vi "EllipseDetection.vi"(0 "Motor an?":bool=TRUE, 1 "Sweep":dbl[](array[numeric])=array[10000 elements], 2 "Winkel_ende":dbl=0.982793723247329, 4 "Sequenz length us":i32=10000, 5 "x_Ellipse":i32=110, 6 "Schrittweite (°)":dbl=1.8 min=0.8999999761581421 max=180.0 step=0.1) -> (7 "Gaparray":dbl[](array[numeric])=[0.0, 0.0, 0.0, 0.0, 0.0, 0.0, 0.0, 0.0, 31.78266847459895, 71.77897962111933, 69.81599676332462, 70.62742631416654, 70.53536343963606, 70.80018094433717, 71.92808960208231, 73.2443285987772, 73.64080618998037, 74.55555718210849], 8 "Max. Index":i32=17, 10 "Maximale Gap":dbl=74.55555718210849, 11 "Wahrscheinlichkeit*Apulitude":dbl[](array[numeric])=[0.0, 0.0, 0.0, 0.0, 0.0, 0.0, 0.0, 0.0, 4.587844159843566e-180, 5.197567004295835, 0.18885512712583885, 1.8492331967600593, 3.0203550412227926, 8.509948855746485, 82.25615517554286, 367.57708439761143, 518.7343556046903, 579.1392161246325], 12 "IR with theshold":dbl[][](graph), 13 "Maximale Gap gefunde?":bool, 14 "Welche Mikrofon arbeitet":tag="Dev2/ai2", 15 "Welche LS arbeitet":i32=4, 16 "Abstatnd":dbl, 17 "Peak Locations":dbl[](array[numeric])=[1600.9324970830344, 1675.4880542651429], 18 "Gap":dbl=74.55555718210849, 19 "Wahrscheinlichkeit":dbl=0.25453954610461715)   [LabVIEW 2014]
uses:
  <vilib>/Analysis/NI_AALBase.lvlib
  <vilib>/Analysis/3filter.llb/Filter Passband Type.ctl
  <vilib>/Analysis/NI_AALPro.lvlib
  <vilib>/Analysis/2dsp.llb/1D Cross Correlation (DBL).vi
  <vilib>/Analysis/3filter.llb/Butterworth Filter (DBL).vi
  <vilib>/Instr/_visa.llb/VISA Configure Serial Port (Instr).vi
panel:
  in  "Registerkarte":T1(tab)=enum."Gap & Wahrscheinlickeit"
  out "Sweep-signal":dbl[](graph)
  out "Anzahl\nMessungen":dbl=18.21266317958185
  in  "Motorwahl":string(combo)="0"
  in  "Stromstärke in mA / 10":u8=40 max=200 step=1
  in  "Schrittgeschwindigkeit":u8=20
  out "time at begin":timestamp=timestamp(3560686964.139921 s since 1904-01-01)
  in  "RN-Motor - RS232":refnum<visa-resource-name>="COM5"
  out "Active Speaker":bool[](array[boolean])=[FALSE, FALSE, FALSE, TRUE, FALSE, FALSE, FALSE, FALSE, FALSE, FALSE, FALSE, FALSE, FALSE, FALSE]
  out "drehrichtung":u8=1
  out "Rohdaten Mic_1":dbl[](graph)
  in  "begin signal":dbl=10000.0
  out "Korreliertes Signal mit richtigem Anfang -M1":dbl[](graph)
  out "Mit Sweep korreliert 1":dbl[](graph)
  in  "Noise Level":dbl=4.0
  in  "RMS miutiplication factor":dbl=3.0
  in  "MaxtPeak miltiplication factor":dbl=7.0
  in  "Grenz Ampulitude":dbl=80.0
  in  "StandardGap":dbl=75.0
  in  "Sigma in Prozent":dbl=2.0
  out "t_2":dbl=1675.4880542651429
  out "t_1":dbl=1600.9324970830344
  out "W * A":dbl=579.1392161246325
  out "Wahrschwinlichkeitsarray":dbl[](array[numeric])=[0.0, 0.0, 0.0, 0.0, 0.0, 0.0, 0.0, 0.0, 1.4779650144959823e-181, 0.026517429714331527, 0.0006779892682999901, 0.003798460831457268, 0.0031702188135415243, 0.005278750347818211, 0.032665581582708055, 0.1340721173746843, 0.17641101202507742, 0.25453954610461715]
  out "Max. Wert":dbl=579.1392161246325
  out "W *A-1":dbl[](array[numeric])=[0.0, 0.0, 0.0, 0.0, 0.0, 0.0, 0.0, 0.0, 4.587844159843566e-180, 5.197567004295835, 0.18885512712583885, 1.8492331967600593, 3.0203550412227926, 8.509948855746485, 82.25615517554286, 367.57708439761143, 518.7343556046903, 579.1392161246325]
  out "GapArray -1":dbl[](array[numeric])=[0.0, 0.0, 0.0, 0.0, 0.0, 0.0, 0.0, 0.0, 31.78266847459895, 71.77897962111933, 69.81599676332462, 70.62742631416654, 70.53536343963606, 70.80018094433717, 71.92808960208231, 73.2443285987772, 73.64080618998037, 74.55555718210849]
  out "t1 Array":dbl[](array[numeric])=[0.0, 0.0, 0.0, 0.0, 0.0, 0.0, 0.0, 0.0, 1194.5330720667082, 1555.0449407198062, 1560.1513249404838, 1564.0418298861218, 1569.529647486898, 1575.4886309745948, 1581.693370955709, 1587.7292742626732, 1594.4280385114012, 1600.9324970830344]
  out "x_Ellipse>100":bool=TRUE
  # "0=links\n1=rechts"
  # "M1: ai2\nM2: ai1"
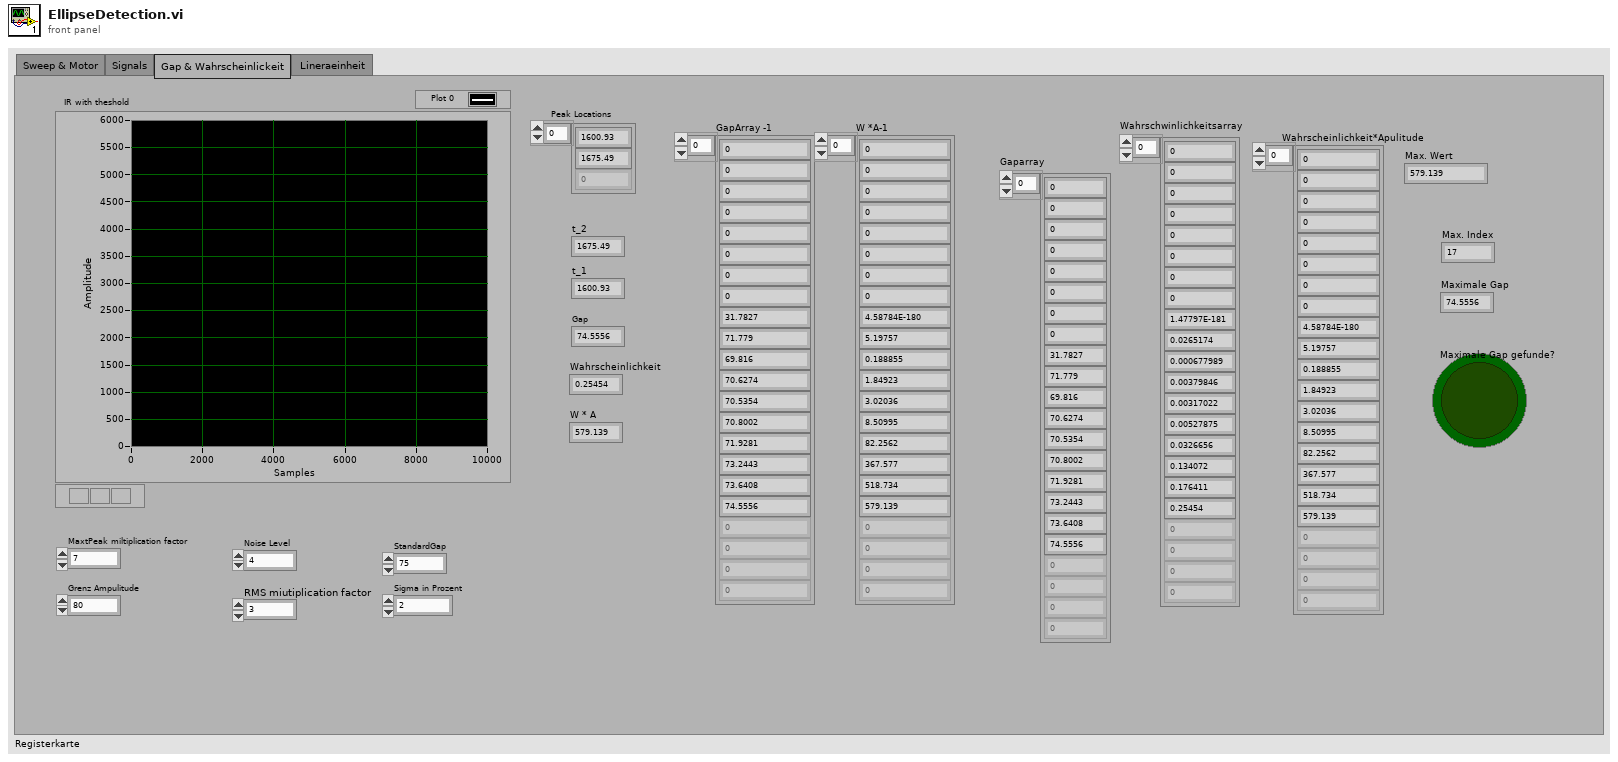
[diagram p1: front panel]
types:
  T1 = enum32{"Sweep & Motor", "Signals", "Gap & Wahrscheinlickeit", "Lineraeinheit "}
  T2 = cluster{"VISA resource name out":refnum<visa-resource-name>, "Motorwahl":string, "Schrittweite (°)":dbl, "error out":errorcluster}
  T3 = cluster{"VISA resource name out":refnum<visa-resource-name>, "Gesendeter Code":string, "Schrittweite (°)":dbl, "error out":errorcluster}
  T4 = typedef "NI_AALBase.lvlib/Filter Passband Type.ctl" = enum32{"Lowpass", "Highpass", "Bandpass", "Bandstop"}
  T5 = cluster{"VISA resource name out":refnum<visa-resource-name>, "Gesendeter Code":string, "error out":errorcluster}
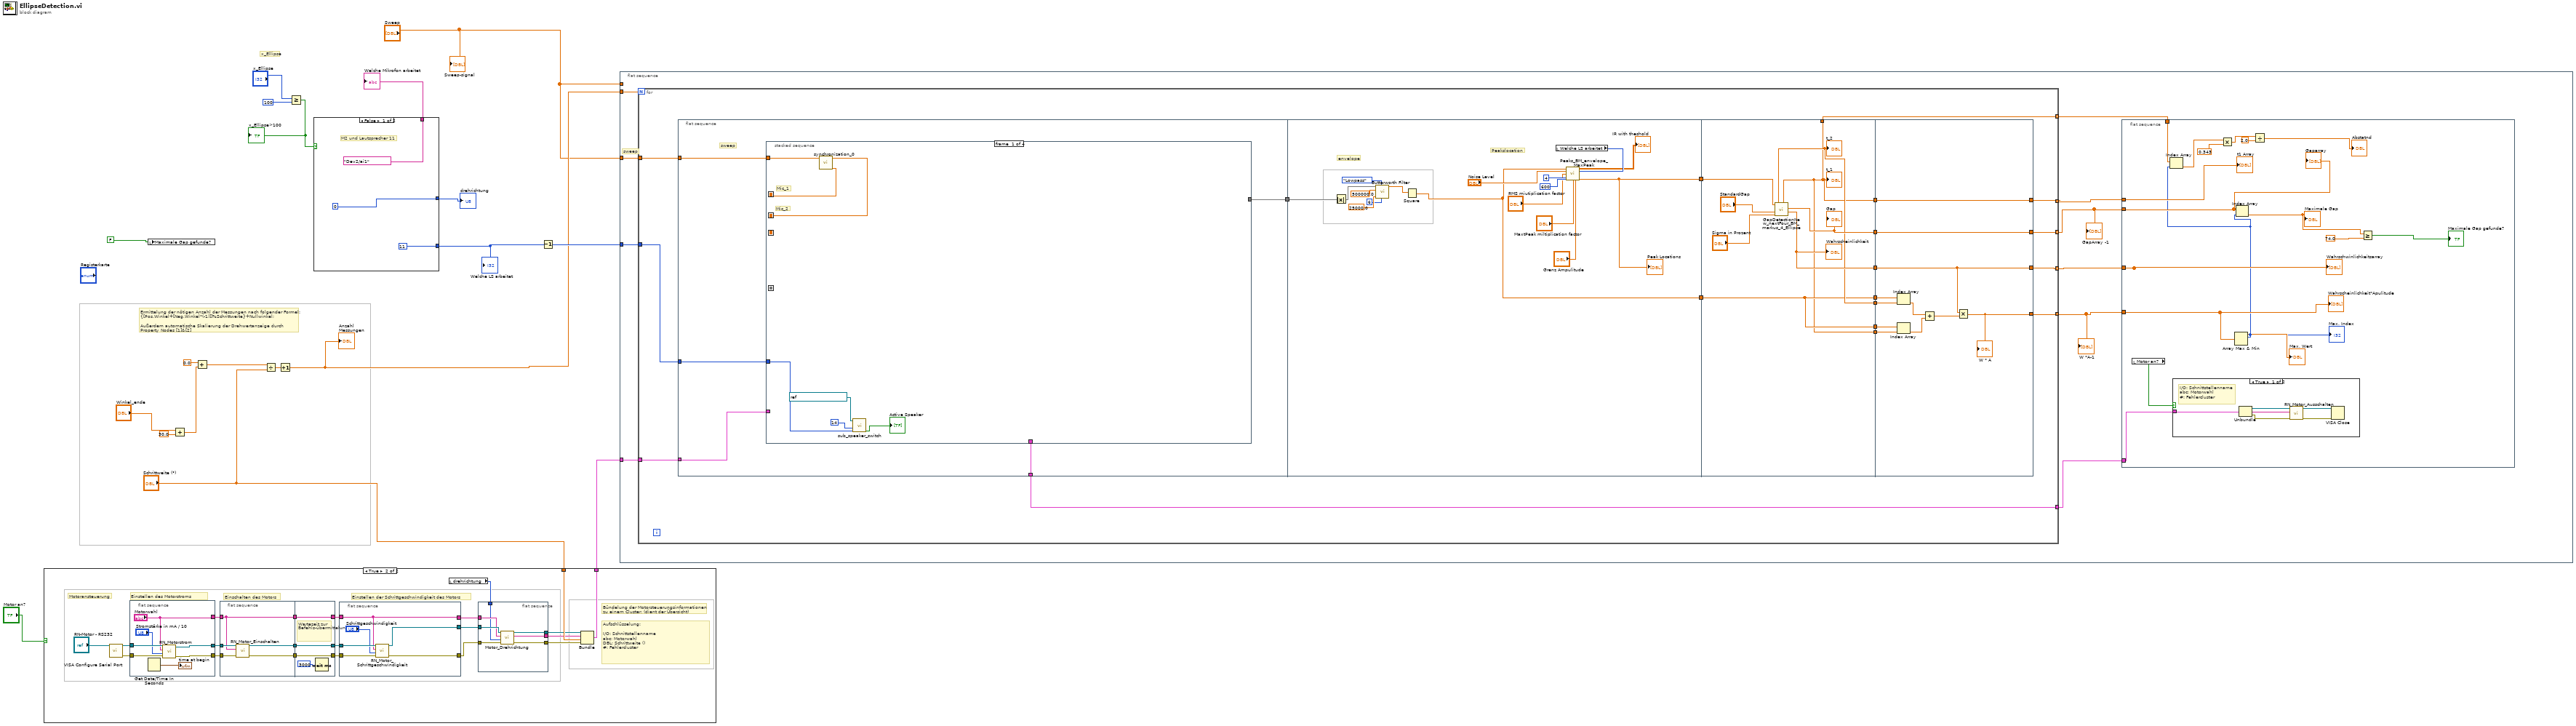
[diagram p0: block diagram]
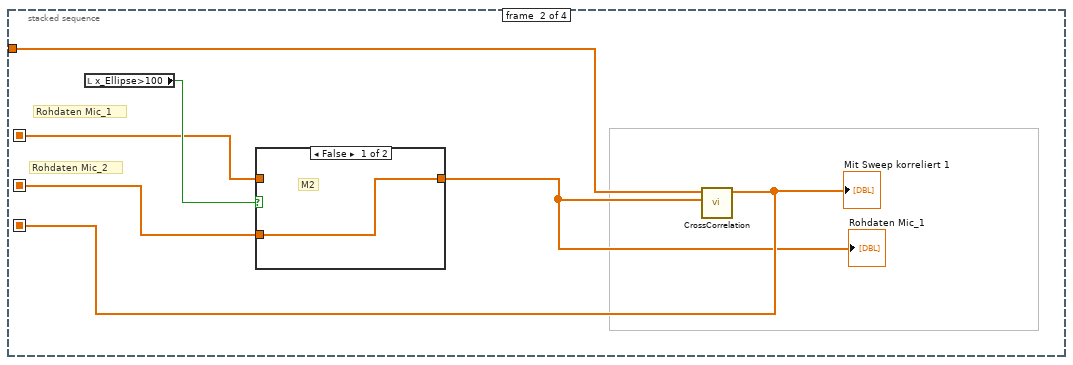
[diagram p3: hidden frame]
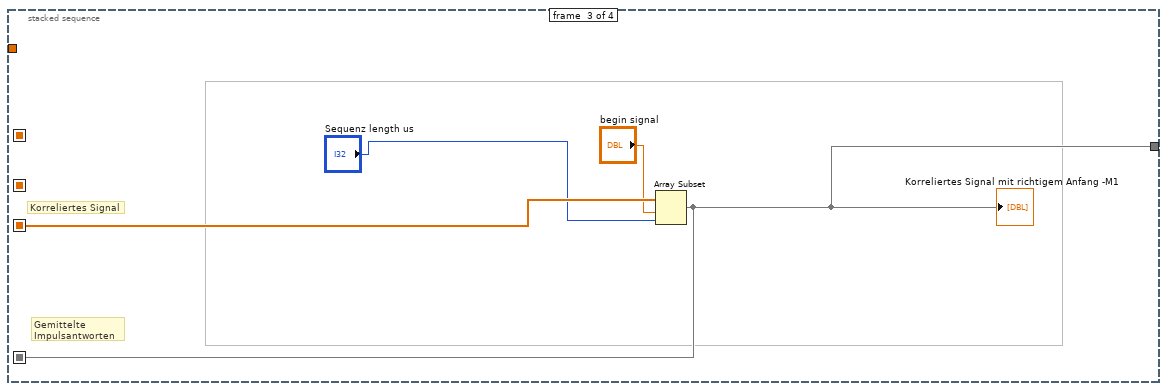
[diagram p5: hidden frame]
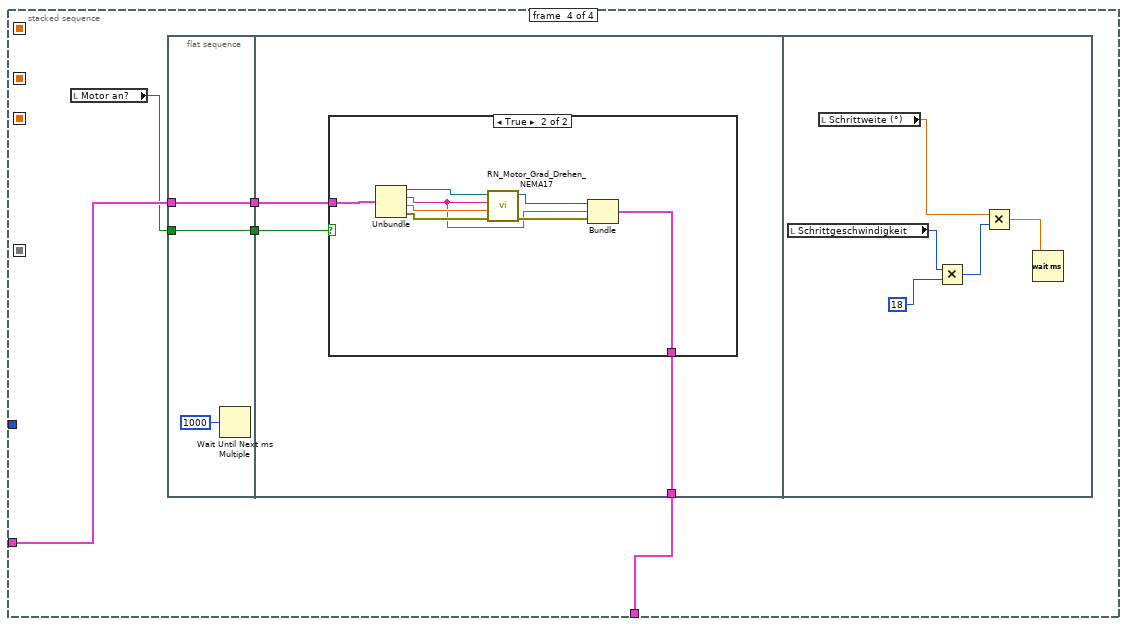
[diagram p6: hidden frame]
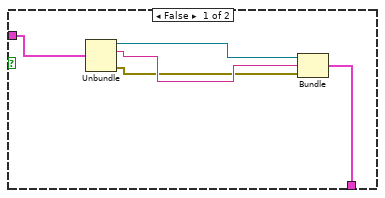
[diagram p7: hidden frame]
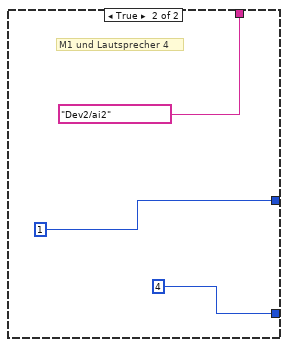
[diagram p8: hidden frame]
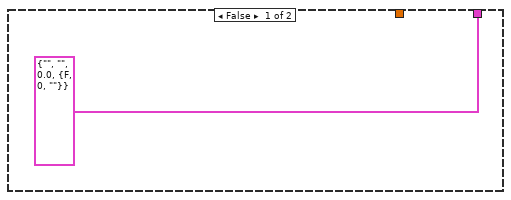
[diagram p9: hidden frame]
diagram:
  # "x_Ellipse"
  # "Ermittelung der nötigen Anzahl der Messungen nach folgender Formel:\n{[Pos.Winkel+[Neg.Winkel*(-1)]]%Schrittweite}+Nullwinkel;\n\nAußerdem automatische Skalierung der Drehwertanzeige durch \nProperty Nodes [1]&[2]"
  n1 = case shown="True" "Motor an?" {
    tunnel: "Schrittweite (°)" -> [_ w29]
    tunnel: [T2 {"VISA resource name out"="", "Motorwahl"="", "Schrittweite (°)"=0.0, "error out"={"status"=FALSE, "code"=0, "source"=""}} ("output cluster") w28] -> w17
    frame False {
    }
    frame True {
      # "Aufschlüsselung:\n\nI/O: Schnittstellenname\nabc: Motorwahl \nDBL: Schrittweite ()\n#: Fehlercluster"
      # "Bündelung der Motorsteuerungsinformationen \nzu einem Cluster: (dient der Übersicht)"
      # "Einstellen der Schrittgeschwindigkeit des Motors"
      # "Einschalten des Motors"
      # "Einstellen des Motorstroms"
      # "Motoransteuerung"
      n2 = call-poly "VISA Configure Serial Port"("VISA resource name"="RN-Motor - RS232") -> ("VISA resource name out"=w37:refnum<visa-resource-name>, "error out"=w36:errorcluster)  [unwired: 13 in]
      n3 = flat-sequence {
        tunnel: w37 -> [w70]
        tunnel: w36 -> [w69]
        tunnel: [w67] -> w35
        tunnel: [w66] -> w34
        tunnel: ["Motorwahl"] -> w30
        frame #0 {
          n4 = Get Date/Time In Seconds() -> (seconds since 1Jan1904=→"time at begin":timestamp)
          n5 = call "RN_Motorstrom.vi"("error in"=w69, "Stromstärke in mA / 10"="Stromstärke in mA / 10", "Motorwahl"="Motorwahl", "VISA resource name in"=w70) -> ("error out"=w66:errorcluster, "VISA resource name out"=w67:refnum<visa-resource-name>)  [unwired: 3 in, 1 out]
        }
      }
      n6 = flat-sequence {
        tunnel: w35 -> [w59]
        tunnel: w34 -> [w58]
        tunnel: w30 -> [w55]
        tunnel: [w57] -> w41
        tunnel: [w56] -> w40
        tunnel: [w55] -> w39
        tunnel: [w62] -> w32
        tunnel: [w63] -> w33
        tunnel: w41 -> [w63]
        tunnel: w40 -> [w62]
        tunnel: [w60] -> w31
        tunnel: w39 -> [w60]
        frame #0 {
          n7 = call "RN_Motor_Einschalten.vi"("error in"=w58, "Motorwahl"=w55, "VISA resource name in"=w59) -> ("error out"=w56:errorcluster, "VISA resource name out"=w57:refnum<visa-resource-name>)  [unwired: 3 in, 2 out]
        }
        frame #1 {
          # "Wartezeit zur Befehls-übermittelung"
          n8 = Wait (ms)(milliseconds to wait=u32 3000) -> ()  [unwired: 1 out]
        }
      }
      n9 = flat-sequence {
        tunnel: w33 -> [w54]
        tunnel: w32 -> [w53]
        tunnel: [w51] -> w27
        tunnel: w31 -> [w50]
        tunnel: [w50] -> w23
        tunnel: [w49] -> w25
        frame #0 {
          n10 = call "RN_Motor_Schrittgeschwindigkeit.vi"("error in"=w53, "Schrittgeschwindigkeit"="Schrittgeschwindigkeit", "Motorwahl"=w50, "VISA resource name in"=w54) -> ("error out"=w51:errorcluster, "VISA resource name out"=w49:refnum<visa-resource-name>)  [unwired: 3 in, 1 out]
        }
      }
      n11 = local read "drehrichtung"() -> (w21:u8)
      n12 = flat-sequence {
        tunnel: w27 -> [w48]
        tunnel: [w47] -> w26
        tunnel: w25 -> [w46]
        tunnel: [w45] -> w24
        tunnel: w23 -> [w44]
        tunnel: [w43] -> w22
        tunnel: w21 -> [w42]
        frame #0 {
          n13 = call "Motor_Drehrichtung.vi"("error in"=w48, "drehrichtung"=w42, "Motorwahl"=w44, "VISA resource name in"=w46) -> ("error out"=w47:errorcluster, "Gesendeter Code"=w43:string, "VISA resource name out"=w45:refnum<visa-resource-name>)  [unwired: 5 in]
        }
      }
      n14 = Bundle("VISA resource name out"=w24, "Gesendeter Code"=w22, "Schrittweite (°)"=w29, "error out"=w26) -> (w28:T3)  [unwired: 1 in]
    }
  }
  n15 = local write "Maximale Gap gefunde?"(FALSE ("Maximale Gap gefunde?")) -> ()
  n16 = Add(x="Winkel_ende", y=30.0) -> (x+y=w3:dbl)
  n17 = Add(x=0.0, y=w3) -> (x+y=w18:dbl)
  n18 = Divide(x=w18, y="Schrittweite (°)") -> (x/y=w19:dbl)
  n19 = Increment(x=w19) -> (x+1=w8:dbl)
  "Anzahl\nMessungen" <- w8
  n20 = Greater Or Equal?(x="x_Ellipse", y=100) -> (x >= y?=w12:bool)
  "x_Ellipse>100" <- w12
  n21 = case shown="False" w12 {
    tunnel: [11 ("Num of Speakers") 4 ("y")] -> w10
    tunnel: [tag "Dev2/ai1" ("physical channels 2") tag "Dev2/ai2" ("physical channels 2")] -> w13
    tunnel: [0 1] -> w6
    frame False {
      # "M2 und Lautsprecher 11"
    }
    frame True {
      # "M1 und Lautsprecher 4"
    }
  }
  "Welche Mikrofon arbeitet" <- w13
  "Welche LS arbeitet" <- w10
  "drehrichtung" <- w6
  n22 = Decrement(x=w10) -> (x-1=w9:i32)
  n23 = flat-sequence {
    tunnel: w8 -> [w86]
    tunnel: w17 -> [w85]
    tunnel: "Sweep" -> [w84]
    tunnel: w9 -> [w83]
    tunnel: "Sweep" -> [_]
    frame #0 {
      # "sweep"
      n24 = for {
        N: w86 -> [_]
        tunnel: w84 -> [w128]
        tunnel: w85 -> [w127]
        tunnel: w83 -> [w125]
        tunnel: [w124] -> w80
        tunnel: [w114] -> w81 mode=indexing
        tunnel: [w122] -> w79 mode=indexing
        tunnel: [w112] -> w82 mode=indexing
        tunnel: [w111] -> w78 mode=indexing
        tunnel: [w110] -> w77 mode=indexing
        n25 = flat-sequence {
          tunnel: w127 -> [w132]
          tunnel: [w131] -> w124
          tunnel: [w130] -> w126
          tunnel: w128 -> [w133]
          tunnel: w125 -> [w129]
          tunnel: w126 -> [w184]
          tunnel: [w183] -> w123
          tunnel: [w182] -> w121
          tunnel: w123 -> [w206]
          tunnel: w121 -> [w200]
          tunnel: [w202] -> w120
          tunnel: [w203] -> w119
          tunnel: [w200] -> w118
          tunnel: [w201] -> w117
          tunnel: [w200] -> w116
          tunnel: [w199] -> w115
          tunnel: [w199] -> w113
          tunnel: [w199] -> w110
          tunnel: [w217] -> w122
          tunnel: [w209] -> w111
          tunnel: w120 -> [w209]
          tunnel: w119 -> [w217]
          tunnel: w118 -> [w214]
          tunnel: w117 -> [w215]
          tunnel: w116 -> [w213]
          tunnel: w115 -> [w212]
          tunnel: [w208] -> w114
          tunnel: [w207] -> w112
          tunnel: w113 -> [w207]
          frame #0 {
            # "sweep"
            n26 = stacked-sequence {
              seq-local: [w135 _ _ _] -> [_ w143 _ _]
              seq-local: [_ w146 _ _] -> [_ _ w152 _]
              seq-local: [_ _ w151 _] -> [_ _ _ _]
              seq-local: [w134 _ _ _] -> [_ w141 _ _]
              tunnel: [_ _ w151 _] -> w130
              tunnel: w133 -> [w137 w145 _ _]
              tunnel: w129 -> [w136 _ _ _]
              tunnel: w132 -> [_ _ _ w157]
              tunnel: [_ _ _ w155] -> w131
              frame #0 {
                # "Mic_2"
                # "Mic_1"
                n27 = call "synchronization_0.vi"("sweep signal"=w137) -> ("Micro 1/ ai 2"=w135:dbl[], "Micro 2/ai 1"=w134:dbl[])  [unwired: 9 in]
                n28 = call "sub_speaker_switch.vi"("Active Speaker\n(Index)"=w136, "Num of Speakers"=14, "task in"=refnum<k21> "Digital_14") -> ("Array (Ausgang)"=→"Active Speaker":bool[])  [unwired: 8 in]
              }
              frame #1 {
                # "Rohdaten Mic_2"
                # "Rohdaten Mic_1"
                n29 = local read "x_Ellipse>100"() -> (w144:bool)
                n30 = case shown="False" w144 {
                  tunnel: w143 -> [_ w148]
                  tunnel: [w147 w148] -> w142
                  tunnel: w141 -> [w147 _]
                  frame False {
                    # "M2"
                  }
                  frame True {
                    # "Mic_1"
                  }
                }
                "Rohdaten Mic_1" <- w142
                n31 = call-poly <vilib>:"CrossCorrelation.vi"("Y"=w142, "X"=w145) -> ("Rxy"=w146:dbl[])  [unwired: 8 in, 1 out]
                "Mit Sweep korreliert 1" <- w146
              }
              frame #2 {
                # "Gemittelte\nImpulsantworten"
                # "Korreliertes Signal"
                n32 = Array Subset(array=w152, index="begin signal", length="Sequenz length us") -> (w151:dbl[])
                "Korreliertes Signal mit richtigem Anfang -M1" <- w151
              }
              frame #3 {
                n33 = local read "Motor an?"() -> (w156:bool)
                n34 = flat-sequence {
                  tunnel: w156 -> [w159]
                  tunnel: w157 -> [w160]
                  tunnel: [w160] -> w154
                  tunnel: [w159] -> w153
                  tunnel: [w161] -> w155
                  tunnel: w154 -> [w163]
                  tunnel: w153 -> [w162]
                  frame #0 {
                    n35 = Wait Until Next ms Multiple(millisecond multiple=u32 1000) -> ()  [unwired: 1 out]
                  }
                  frame #1 {
                    n36 = case shown="True" w162 {
                      tunnel: w163 -> [w167 w176]
                      tunnel: [w164 w169] -> w161
                      frame False {
                        n37 = Unbundle(w167) -> ("VISA resource name out"=w166:refnum<visa-resource-name>, "Gesendeter Code"=w168:string, "error out"=w165:errorcluster)  [unwired: 1 out]
                        n38 = Bundle("VISA resource name out"=w166, "Gesendeter Code"=w168, "error out"=w165) -> (w164:T5)  [unwired: 1 in]
                      }
                      frame True {
                        n39 = Unbundle(w176) -> ("VISA resource name out"=w175:refnum<visa-resource-name>, "Gesendeter Code"=w170:string, "Schrittweite (°)"=w173:dbl, "error out"=w172:errorcluster)
                        n40 = call "RN_Motor_Grad_Drehen_NEMA17.vi"("error in"=w172, "Drehwinkel (°)"=w173, "Motorwahl"=w170, "VISA resource name in"=w175) -> ("error out"=w171:errorcluster, "VISA resource name out"=w174:refnum<visa-resource-name>)  [unwired: 3 in, 1 out]
                        n41 = Bundle("VISA resource name out"=w174, "Gesendeter Code"=w170, "error out"=w171) -> (w169:T5)  [unwired: 1 in]
                      }
                    }
                  }
                  frame #2 {
                    n42 = local read "Schrittgeschwindigkeit"() -> (w177:u8)
                    n43 = local read "Schrittweite (°)"() -> (w179:dbl)
                    n44 = Multiply(x=w177, y=u32 18 ("milliseconds to wait")) -> (x*y=w181:u32)
                    n45 = Multiply(x=w179, y=w181) -> (x*y=w180:dbl)
                    n46 = Wait (ms)(milliseconds to wait=w180) -> ()  [unwired: 1 out]
                  }
                }
              }
            }
          }
          frame #1 {
            # "Peakslocation"
            # "envelope"
            n47 = Absolute Value(x=w184) -> (abs(x)=w194:dbl[])
            n48 = call-poly <vilib>:"Butterworth Filter.vi"("order"=6, "filter type"=Filter_Passband_Type."Lowpass", "low cutoff freq: fl"=25000.0 ("high cutoff freq: fh"), "sampling freq: fs"=500000.0, "X"=w194) -> ("Filtered X"=w193:dbl[])  [unwired: 3 in, 1 out]
            n49 = Square(x=w193) -> (x^2=w182:dbl[])
            n50 = local read "Welche LS arbeitet"() -> (w186:i32)
            n51 = call "Peaks_BM_envelope_MaxPeak.vi"("imput sequence"=w182, "Noise Level"="Noise Level", "welche LS ?"=w186, "RMS miutiplication factor"="RMS miutiplication factor", "width 1"=4 ("width"), "Length of Lsimp"=600, "MaxPeak miltiplication factor"="MaxtPeak miltiplication factor", "Grenz Ampulitude"="Grenz Ampulitude") -> ("IR with theshold"=→"IR with theshold":dbl[][], "Peak Locations"=w183:dbl[])  [unwired: 5 in, 1 out]
            "Peak Locations" <- w183
          }
          frame #2 {
            n52 = call "GapDetectionNew_nextFour_BM_markus_4_Ellipse.vi"("Sigma in Prozent"="Sigma in Prozent", "Gap"="StandardGap", "Locations"=w206) -> ("Wahrscheinlichkeit"=w202:dbl, "Gap"=w203:dbl, "t_1"=w199:dbl, "t_2"=w201:dbl)  [unwired: 4 in, 1 out]
            "Gap" <- w203
            "Wahrscheinlichkeit" <- w202
            "t_2" <- w201
            "t_1" <- w199
          }
          frame #3 {
            n53 = Index Array(array=w214, index=w215) -> (element=w211:dbl)
            n54 = Index Array(array=w213, index=w212) -> (element=w216:dbl)
            n55 = Add(x=w211, y=w216) -> (x+y=w210:dbl)
            n56 = Multiply(x=w209, y=w210) -> (x*y=w208:dbl)
            "W * A" <- w208
          }
        }
      }
      "GapArray -1" <- w79
      "W *A-1" <- w81
      n57 = flat-sequence {
        tunnel: w82 -> [w101]
        tunnel: w81 -> [w98]
        tunnel: w80 -> [w102]
        tunnel: w79 -> [w100]
        tunnel: [w99] -> _
        tunnel: w78 -> [w99]
        tunnel: w77 -> [w93]
        frame #0 {
          n58 = local read "Motor an?"() -> (w103:bool)
          n59 = case shown="True" w103 {
            tunnel: w102 -> [w104 _]
            frame True {
              # "I/O: Schnittstellenname\nabc: Motorwahl \n#: Fehlercluster"
              n60 = Unbundle(w104) -> ("VISA resource name out"=w107:refnum<visa-resource-name>, "Gesendeter Code"=w106:string, "error out"=w105:errorcluster)
              n61 = call "RN_Motor_Ausschalten.vi"("error in"=w105, "Motorwahl"=w106, "VISA resource name in"=w107) -> ("error out"=w108:errorcluster, "VISA resource name out"=w109:refnum<visa-resource-name>)  [unwired: 3 in, 2 out]
              n62 = VISA Close(VISA resource name=w109, error in (no error)=w108) -> ()  [unwired: 1 out]
            }
            frame False {
            }
          }
          n63 = Array Max & Min(array=w98) -> (max value=→"Max. Wert":dbl, max index (indices)=w92:i32)  [unwired: 2 out]
          "Max. Index" <- w92
          n64 = Index Array(array=w93, index=w92) -> (element=w91:dbl)
          n65 = Multiply(x=w91, y=0.343) -> (x*y=w89:dbl)
          n66 = Index Array(array=w100, index=w92) -> (element=w96:dbl)
          "Maximale Gap" <- w96
          n67 = Divide(x=w89, y=2.0) -> (x/y=→"Abstatnd":dbl)
          n68 = Greater Or Equal?(x=w96, y=74.0) -> (x >= y?=→"Maximale Gap gefunde?":bool)
          "t1 Array" <- w101
          "Gaparray" <- w100
          "Wahrschwinlichkeitsarray" <- w99
          "Wahrscheinlichkeit*Apulitude" <- w98
        }
      }
    }
  }
  "Sweep-signal" <- "Sweep"
